vi "Read File.vi"(8 "error in":errorcluster, 11 "ITX":refnum<class "Data.ITX.lvclass">) -> (0 "error out":errorcluster, 3 "ITX out":refnum<class "Data.ITX.lvclass">)   [LabVIEW 2016, in "Data.ITX.lvclass"]
uses:
  Data.ITX.lvclass
  C:/user/patrick/git/LV-to-ITX/src/Data/Data.lvclass
  Data/Data.lvclass/Data.ctl
  Data/Data.lvclass
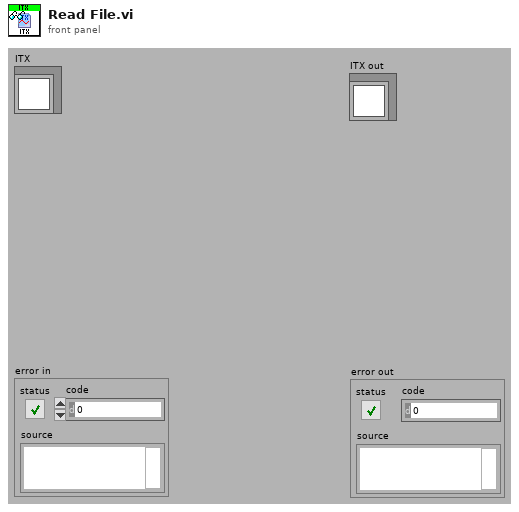
[diagram p1: front panel]
types:
  T1 = typedef "Data.lvclass/Dictionary--cluster.ctl" = cluster{"key":string, "value":variant}
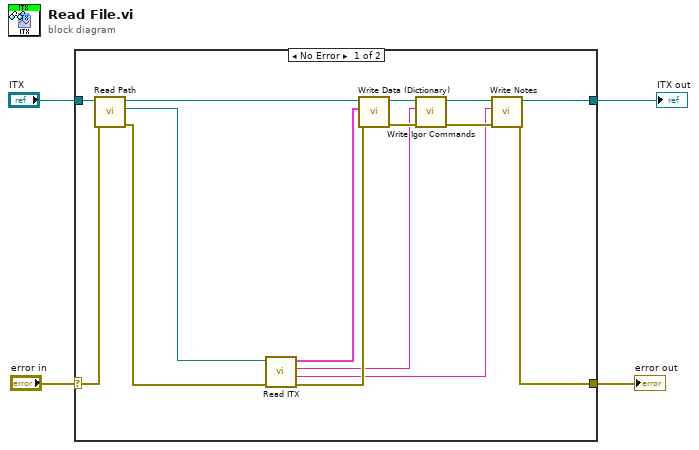
[diagram p0: block diagram]
diagram:
  n1 = case shown="No Error" "error in" {
    selector: "error in" -> [w6 w21]
    tunnel: "ITX" -> [w19 w20]
    tunnel: [w18 w20] -> w3
    tunnel: [w12 w21] -> w2
    frame No Error {
      n2 = call "Read Path.vi"("error in (no error)"=w6, "Data Save"=w19) -> ("error out"=w11:errorcluster, "Path"=w5:path, "Data Save out"=w15:refnum<class "Data.ITX.lvclass">)  [unwired: 7 in]
      n3 = call "Read ITX.vi"("error in (no error)"=w11, "Path"=w5) -> ("error out"=w10:errorcluster, "Commands"=w7:string, "Notes"=w8:string, "Data (Dictionary)"=w9:T1[])  [unwired: 6 in]
      n4 = call "Write Data (Dictionary).vi"("error in (no error)"=w10, "Data (Dictionary)"=w9, "Data Save"=w15) -> ("error out"=w14:errorcluster, "Data Save out"=w16:refnum<class "Data.ITX.lvclass">)  [unwired: 7 in]
      n5 = call "Write Igor Commands.vi"("error in (no error)"=w14, "Igor Commands"=w8, "Data Save"=w16) -> ("error out"=w13:errorcluster, "Data Save out"=w17:refnum<class "Data.ITX.lvclass">)  [unwired: 7 in]
      n6 = call "Write Notes.vi"("error in (no error)"=w13, "Notes"=w7, "Data Save"=w17) -> ("error out"=w12:errorcluster, "Data Save out"=w18:refnum<class "Data.ITX.lvclass">)  [unwired: 7 in]
    }
    frame Error {
    }
  }
  "error out" <- w2
  "ITX out" <- w3
